vi "Reset Routine SLM.vi"(11 "Numeric":i32) -> ()   [LabVIEW 2014]
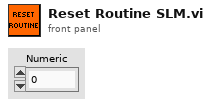
[diagram p1: front panel]
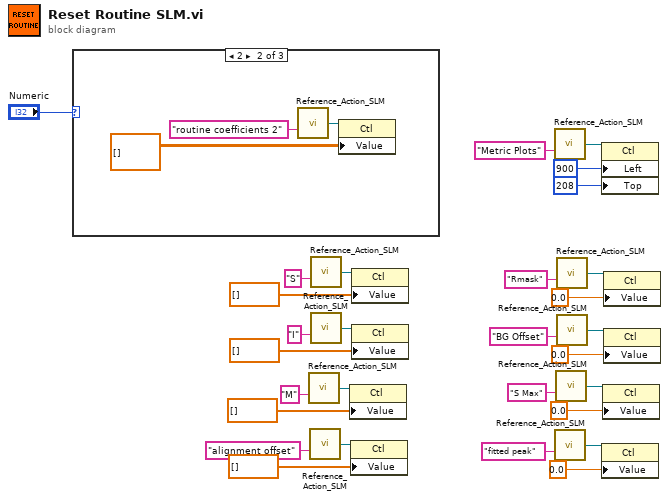
[diagram p0: block diagram]
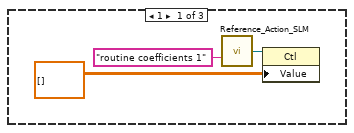
[diagram p2: hidden frame]
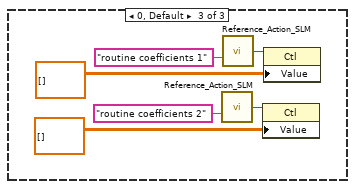
[diagram p3: hidden frame]
diagram:
  n1 = case shown="2" "Numeric" {
    frame 1 {
      n2 = call "Reference_Action_SLM.vi"("Control Name"="routine coefficients 1") -> ("Ref OUT"=w31:refnum<vi>)  [unwired: 12 in, 2 out]
      n3 = property class="Ctl"(reference=w31, "Value"=dbl[][] [] ("Mode Coeffs")) -> ()  [unwired: 1 in, 2 out]
    }
    frame 2 {
      n4 = call "Reference_Action_SLM.vi"("Control Name"="routine coefficients 2") -> ("Ref OUT"=w34:refnum<vi>)  [unwired: 12 in, 2 out]
      n5 = property class="Ctl"(reference=w34, "Value"=dbl[][] [] ("Mode Coeffs")) -> ()  [unwired: 1 in, 2 out]
    }
    frame 0, Default {
      n6 = call "Reference_Action_SLM.vi"("Control Name"="routine coefficients 2") -> ("Ref OUT"=w37:refnum<vi>)  [unwired: 12 in, 2 out]
      n7 = call "Reference_Action_SLM.vi"("Control Name"="routine coefficients 1") -> ("Ref OUT"=w40:refnum<vi>)  [unwired: 12 in, 2 out]
      n8 = property class="Ctl"(reference=w37, "Value"=dbl[][] [] ("Mode Coeffs")) -> ()  [unwired: 1 in, 2 out]
      n9 = property class="Ctl"(reference=w40, "Value"=dbl[][] [] ("Mode Coeffs")) -> ()  [unwired: 1 in, 2 out]
    }
  }
  n10 = call "Reference_Action_SLM.vi"("Control Name"="M") -> ("Ref OUT"=w15:refnum<vi>)  [unwired: 12 in, 2 out]
  n11 = call "Reference_Action_SLM.vi"("Control Name"="alignment offset") -> ("Ref OUT"=w12:refnum<vi>)  [unwired: 12 in, 2 out]
  n12 = call "Reference_Action_SLM.vi"("Control Name"="S") -> ("Ref OUT"=w21:refnum<vi>)  [unwired: 12 in, 2 out]
  n13 = call "Reference_Action_SLM.vi"("Control Name"="I") -> ("Ref OUT"=w18:refnum<vi>)  [unwired: 12 in, 2 out]
  n14 = property class="Ctl"(reference=w15, "Value"=dbl[] [] ("Ab Corr VI.I")) -> ()  [unwired: 1 in, 2 out]
  n15 = property class="Ctl"(reference=w12, "Value"=dbl[] [] ("Ab Corr VI.I")) -> ()  [unwired: 1 in, 2 out]
  n16 = property class="Ctl"(reference=w21, "Value"=dbl[] [] ("Ab Corr VI.I")) -> ()  [unwired: 1 in, 2 out]
  n17 = property class="Ctl"(reference=w18, "Value"=dbl[] [] ("Ab Corr VI.I")) -> ()  [unwired: 1 in, 2 out]
  n18 = call "Reference_Action_SLM.vi"("Control Name"="Metric Plots") -> ("Ref OUT"=w29:refnum<vi>)  [unwired: 12 in, 2 out]
  n19 = call "Reference_Action_SLM.vi"("Control Name"="fitted peak") -> ("Ref OUT"=w25:refnum<vi>)  [unwired: 12 in, 2 out]
  n20 = call "Reference_Action_SLM.vi"("Control Name"="S Max") -> ("Ref OUT"=w10:refnum<vi>)  [unwired: 12 in, 2 out]
  n21 = call "Reference_Action_SLM.vi"("Control Name"="Rmask") -> ("Ref OUT"=w4:refnum<vi>)  [unwired: 12 in, 2 out]
  n22 = call "Reference_Action_SLM.vi"("Control Name"="BG Offset") -> ("Ref OUT"=w7:refnum<vi>)  [unwired: 12 in, 2 out]
  n23 = property on="Property Node" class="Ctl"(reference=w29, "Left"=900 ("Position:Left"), "Top"=208 ("Position:Top")) -> ()  [unwired: 1 in, 2 out]
  n24 = property on="Property Node" class="Ctl"(reference=w25, "Value"=0.0) -> ()  [unwired: 1 in, 2 out]
  n25 = property on="Property Node" class="Ctl"(reference=w10, "Value"=0.0) -> ()  [unwired: 1 in, 2 out]
  n26 = property on="Property Node" class="Ctl"(reference=w4, "Value"=0.0) -> ()  [unwired: 1 in, 2 out]
  n27 = property on="Property Node" class="Ctl"(reference=w7, "Value"=0.0) -> ()  [unwired: 1 in, 2 out]
